vi "S&E text file string header.vi"(9 "error in (no error)":errorcluster, 13 "Delimiter(;)":string=";") -> (6 "Simple Header":string, 8 "Full Header":string, 10 "error out":errorcluster)   [LabVIEW 2011]
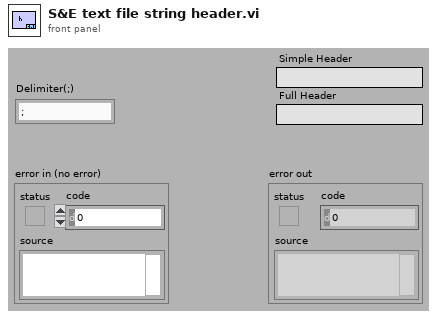
[diagram p1: front panel]
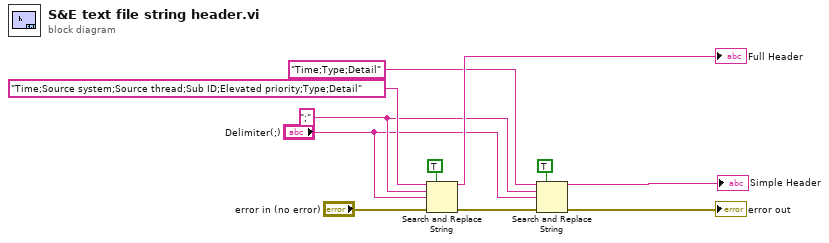
[diagram p0: block diagram]
diagram:
  w4 = ";" ("search string")
  n1 = Search and Replace String(replace all?=TRUE ("replace all? (F)"), input string="Time;Source system;Source thread;Sub ID;Elevated priority;Type;Detail" ("format string"), search string=w4, replace string="Delimiter(;)", error in="error in (no error)") -> (result string=→"Full Header":string, error out=w7:errorcluster)  [unwired: 3 in, 2 out]
  n2 = Search and Replace String(replace all?=TRUE ("replace all? (F)"), input string="Time;Type;Detail" ("format string"), search string=w4, replace string="Delimiter(;)", error in=w7) -> (result string=→"Simple Header":string, error out=→"error out":errorcluster)  [unwired: 3 in, 2 out]
